vi "IsItemRelated.vi"(8 "error in (no error)":errorcluster, 9 "Item to compare":refnum<class "ILabVIEWItem.lvclass">, 11 "CLabVIEWItem in":refnum<class "CLabVIEWItem.lvclass">) -> (0 "error out":errorcluster, 2 "Is item related?":bool, 3 "CLabVIEWItem out":refnum<class "CLabVIEWItem.lvclass">)   [LabVIEW 2020, in "LabVIEWItem.lvlib" / "CLabVIEWItem.lvclass"]
uses:
  CLabVIEWItem.lvclass
  obj/Addons/LabVIEWObjectInterfaces.lvlibp/LabVIEWObjectInterfaces/ILabVIEWItem/ILabVIEWItem.lvclass
  CommonHelpers/CommonHelpers.lvlib
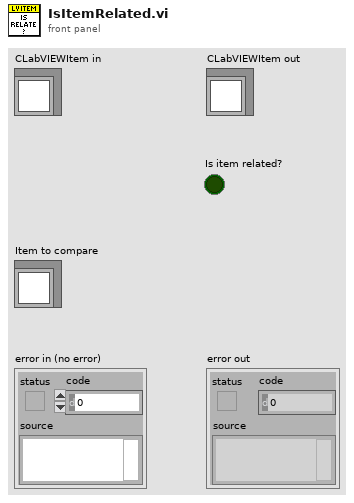
[diagram p1: front panel]
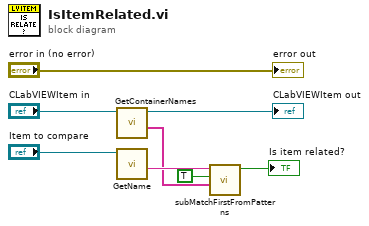
[diagram p0: block diagram]
diagram:
  n1 = call-dynamic "GetContainerNames.vi"("CLabVIEWItem in"="CLabVIEWItem in") -> ("Container name[]"=w5:string[], "CLabVIEWItem out"=→"CLabVIEWItem out":refnum<class "CLabVIEWItem.lvclass">)  [unwired: 8 in, 1 out]
  n2 = call-dynamic "GetName.vi"("ILabVIEWItem in"="Item to compare") -> ("Name"=w6:string)  [unwired: 8 in, 2 out]
  n3 = call "subMatchFirstFromPatterns.vi"("patterns"=w5, "exact match?"=TRUE, "string in"=w6) -> ("found?"=→"Is item related?":bool)  [unwired: 6 in, 2 out]
  "error out" <- "error in (no error)"
